vi "Active Channels controller.vi"(6 "Off delay period (s)":dbl, 7 "Current time":dbl, 8 "Shift In":cluster{"Time ":dbl, "Channel State":bool}, 9 "Channels commencing with these characters":string="EnFlo_Tunnel:Return_Temp:Floor", 10 "Control Channel State":bool, 11 "Control on":T1) -> (0 "Shift Out":cluster{"Time ":dbl, "Channel State":bool})   [LabVIEW 2015]
uses:
  ADAM Client/Sub VIs/Channel_State_Control.ctl
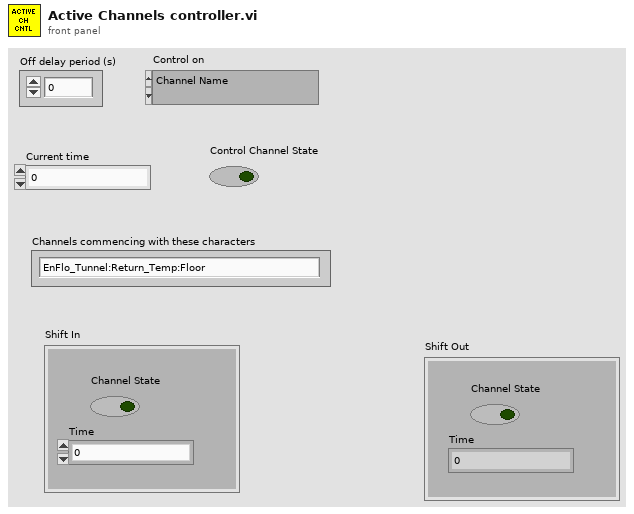
[diagram p1: front panel]
types:
  T1 = typedef "Channel_State_Control.ctl" = enum16{"Channel Name", "Channel Name Starts with", "Main Address"}
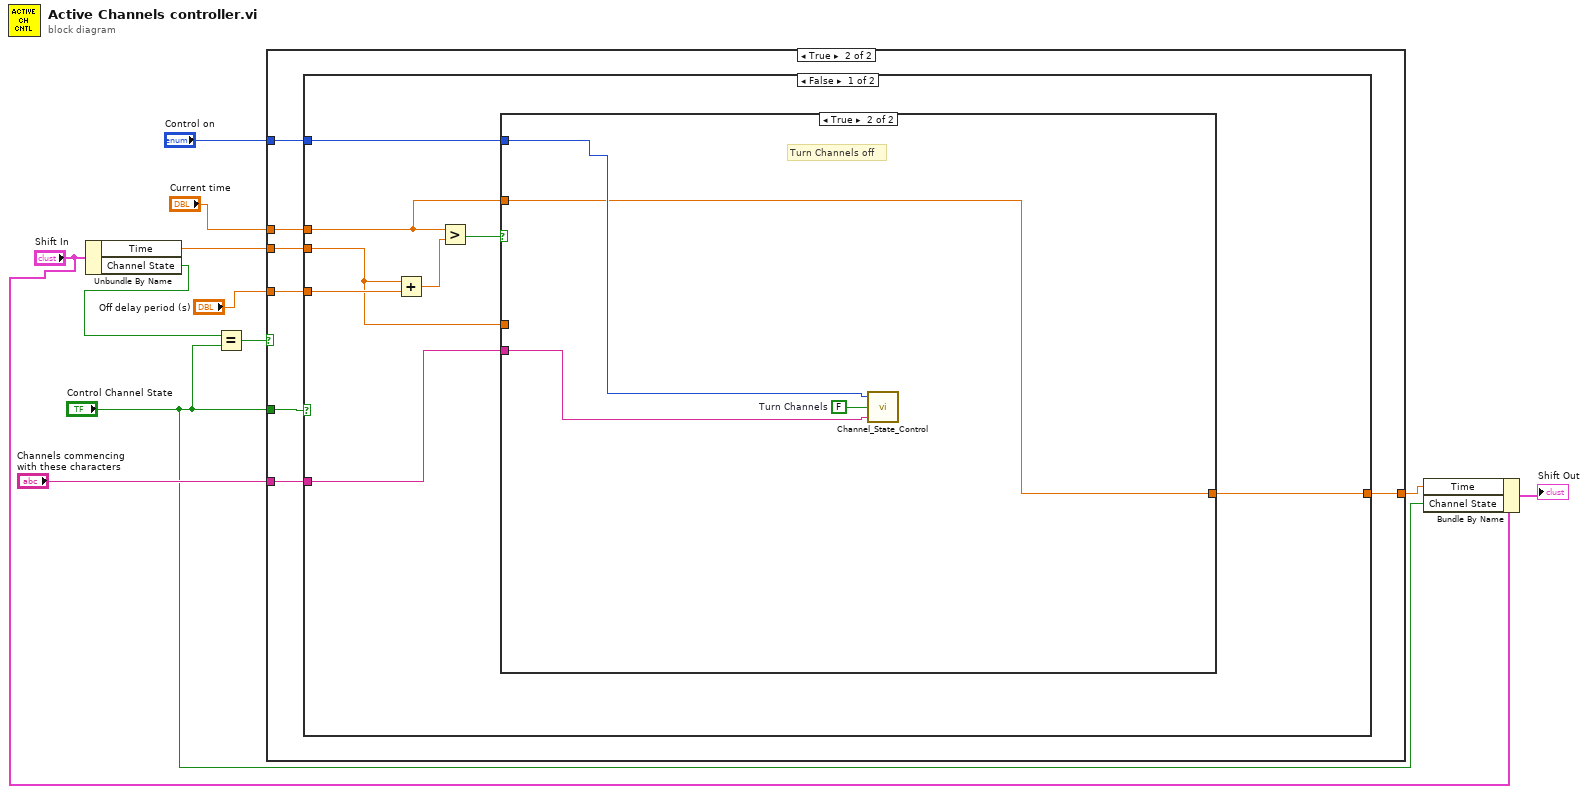
[diagram p0: block diagram]
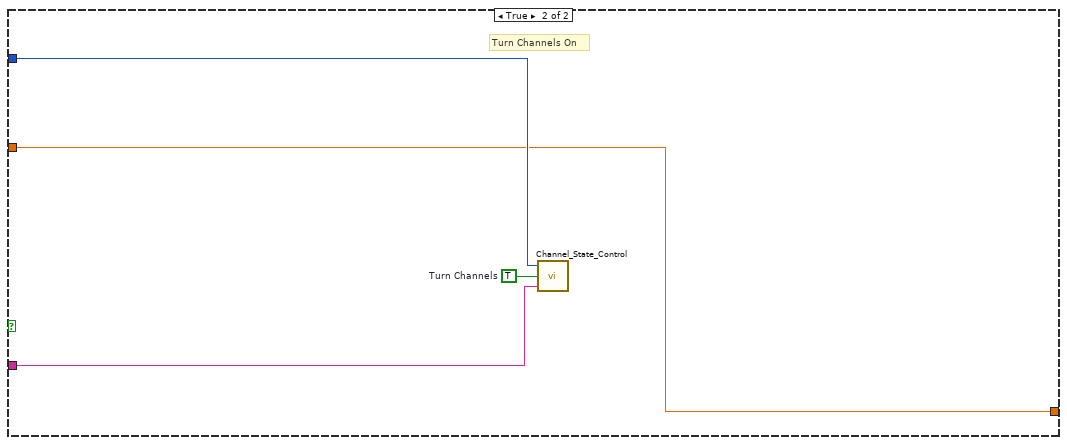
[diagram p3: hidden frame]
diagram:
  n1 = Unbundle By Name("Shift In") -> ("Time"=w6:dbl, "Channel State"=w3:bool)
  n2 = Equal?(x=w3, y="Control Channel State") -> (x = y?=w11:bool)
  n3 = case shown="True" w11 {
    tunnel: "Control Channel State" -> [w16 w28]
    tunnel: "Current time" -> [w14 w27]
    tunnel: w6 -> [_ w26]
    tunnel: "Off delay period (s)" -> [_ w25]
    tunnel: "Channels commencing with these characters" -> [w12 w24]
    tunnel: [w15 w23] -> w4
    tunnel: "Control on" -> [w13 w22]
    frame False {
      n4 = case shown="False" w16 {
        tunnel: [w17 w18] -> w15
        tunnel: w14 -> [w17 w18]
        tunnel: w13 -> [_ w20]
        tunnel: w12 -> [_ w19]
        frame False {
        }
        frame True {
          w21 = TRUE  # Turn Channels
          # "Turn Channels On"
          n5 = call "Channel_State_Control.vi"("Match"=w19, "Turn Channels"=w21, "Control on"=w20) -> ()  [unwired: 2 out]
        }
      }
    }
    frame True {
      n6 = case shown="False" w28 {
        tunnel: w27 -> [w29 _]
        tunnel: w26 -> [w31 w42]
        tunnel: w25 -> [w36 _]
        tunnel: w24 -> [w33 _]
        tunnel: [w32 w42] -> w23
        tunnel: w22 -> [w30 _]
        frame False {
          n7 = Add(x=w31, y=w36) -> (x+y=w35:dbl)
          n8 = Greater?(x=w29, y=w35) -> (0:w34:bool)
          n9 = case shown="True" w34 {
            tunnel: w33 -> [_ w39]
            tunnel: [w37 w38] -> w32
            tunnel: w31 -> [w37 _]
            tunnel: w30 -> [_ w40]
            tunnel: w29 -> [_ w38]
            frame False {
            }
            frame True {
              w41 = FALSE  # Turn Channels
              # "Turn Channels off"
              n10 = call "Channel_State_Control.vi"("Match"=w39, "Turn Channels"=w41, "Control on"=w40) -> ()  [unwired: 2 out]
            }
          }
        }
        frame True {
        }
      }
    }
  }
  n11 = Bundle By Name(cluster="Shift In", "Time"=w4, "Channel State"="Control Channel State") -> (→"Shift Out":cluster{"Time ":dbl, "Channel State":bool})
